vi "wait_for_T_v2.vi"(9 "Toleranz (%)":dbl, 10 "VISA session 2":refnum<visa-resource-name>, 11 "T_target":dbl) -> (2 "dup VISA session":refnum<visa-resource-name>, 3 "T innerhalb Toleranz":bool)   [LabVIEW 2010]
uses:
  Instrument_Setup.vi
panel:
  in  "iter":i32=50
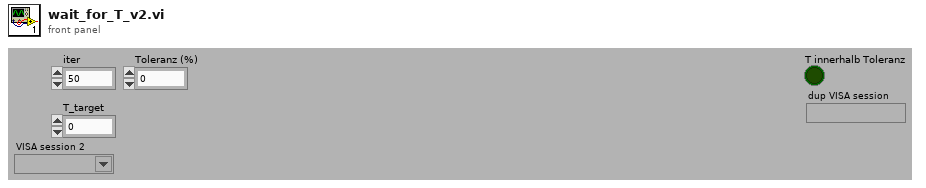
[diagram p1: front panel]
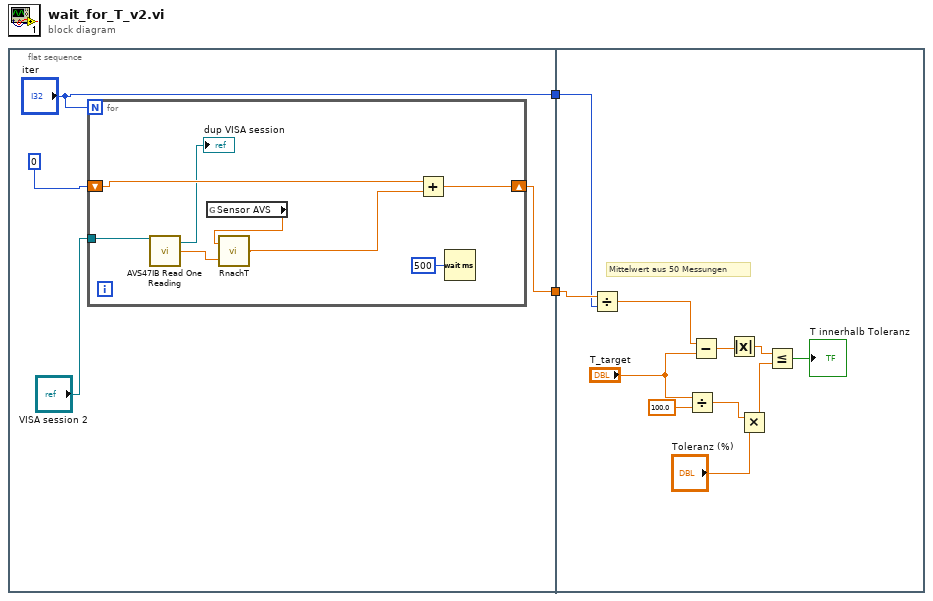
[diagram p0: block diagram]
diagram:
  n1 = flat-sequence {
    tunnel: [w5] -> w2
    tunnel: ["iter"] -> w1
    tunnel: w2 -> [w25]
    tunnel: w1 -> [w24]
    frame #0 {
      n2 = for {
        N: "iter" -> [_]
        shift-right: [w13] -> w5
        shift-left: 0 -> [w14]
        tunnel: "VISA session 2" -> [w7]
        n3 = call "AVS47IB Read One Reading.vi"("VISA session"=w7) -> ("dup VISA session"=→"dup VISA session":refnum<visa-resource-name>, "Resistance reading"=w11:dbl)  [unwired: 10 in, 3 out]
        n4 = global read "Instrument_Setup.vi" "Sensor AVS"() -> (w12:dbl)
        n5 = call "RnachT.vi"("R"=w11, "Sensor Cal #"=w12) -> ("T (K)"=w9:dbl)
        n6 = Add(x=w14, y=w9) -> (x+y=w13:dbl)
        n7 = Wait (ms)(milliseconds to wait=u32 500) -> ()  [unwired: 1 out]
      }
    }
    frame #1 {
      # "Mittelwert aus 50 Messungen"
      n8 = Divide(x=w25, y=w24) -> (x/y=w23:dbl)
      n9 = Divide(x="T_target", y=100.0) -> (x/y=w19:dbl)
      n10 = Subtract(x=w23, y="T_target") -> (x-y=w16:dbl)
      n11 = Absolute Value(x=w16) -> (abs(x)=w15:dbl)
      n12 = Multiply(x=w19, y="Toleranz (%)") -> (x*y=w17:dbl)
      n13 = Less Or Equal?(x=w15, y=w17) -> (x <= y?=→"T innerhalb Toleranz":bool)
    }
  }
